vi "Read_Interlocks.vi"(8 "Error In":errorcluster, 11 "AccelNET.lvlib:TCP.lvclass":refnum<class "TCP.lvclass">) -> (0 "Error Out":errorcluster, 2 "Interlock Status":T1)   [LabVIEW 2012, in "AccelNET.lvlib" / "TCP.lvclass"]
uses:
  TCP.lvclass
  Interlocks.ctl
  Read_Selector.ctl
  Useful_Controls.lvlib
  Useful_SubVIs.lvlib
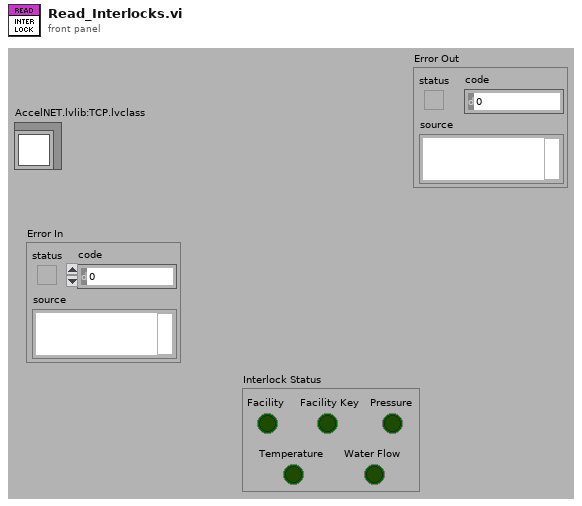
[diagram p1: front panel]
types:
  T1 = typedef "AccelNET.lvlib/Useful_Controls.lvlib/Interlocks.ctl" = cluster{"Facility":bool, "Facility Key":bool, "Water Flow":bool, "Pressure":bool, "Temperature":bool}
  T2 = typedef "AccelNET.lvlib/Useful_Controls.lvlib/Read_Selector.ctl" = u16
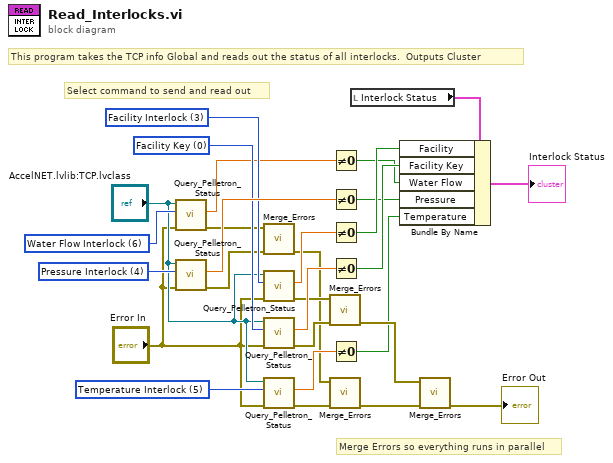
[diagram p0: block diagram]
diagram:
  w20 = T2 5 items=["Facility Key", "Chain Bypass", "Rotating Shaft Bypass", "Facility Interlock", "Pressure Interlock", "Temperature Interlock", "Water Flow Interlock", "Blower Status", "High Voltage", "+ High Voltage PS Readout", "- High Voltage PS Readout", "High Voltage PS Setting", "Ion Gauge", "Ion Filament", "Control Reference Voltage", "Control Mode", "Power Supply", "Chain Current", "Column Current", "Lost Current", "High Voltage Power Supply", "Rotating Shaft", "Chain", "Beamline GV"] ("Read Selector")
  w22 = T2 6 items=["Facility Key", "Chain Bypass", "Rotating Shaft Bypass", "Facility Interlock", "Pressure Interlock", "Temperature Interlock", "Water Flow Interlock", "Blower Status", "High Voltage", "+ High Voltage PS Readout", "- High Voltage PS Readout", "High Voltage PS Setting", "Ion Gauge", "Ion Filament", "Control Reference Voltage", "Control Mode", "Power Supply", "Chain Current", "Column Current", "Lost Current", "High Voltage Power Supply", "Rotating Shaft", "Chain", "Beamline GV"] ("Read Selector")
  w24 = T2 0 items=["Facility Key", "Chain Bypass", "Rotating Shaft Bypass", "Facility Interlock", "Pressure Interlock", "Temperature Interlock", "Water Flow Interlock", "Blower Status", "High Voltage", "+ High Voltage PS Readout", "- High Voltage PS Readout", "High Voltage PS Setting", "Ion Gauge", "Ion Filament", "Control Reference Voltage", "Control Mode", "Power Supply", "Chain Current", "Column Current", "Lost Current", "High Voltage Power Supply", "Rotating Shaft", "Chain", "Beamline GV"] ("Read Selector")
  w26 = T2 3 items=["Facility Key", "Chain Bypass", "Rotating Shaft Bypass", "Facility Interlock", "Pressure Interlock", "Temperature Interlock", "Water Flow Interlock", "Blower Status", "High Voltage", "+ High Voltage PS Readout", "- High Voltage PS Readout", "High Voltage PS Setting", "Ion Gauge", "Ion Filament", "Control Reference Voltage", "Control Mode", "Power Supply", "Chain Current", "Column Current", "Lost Current", "High Voltage Power Supply", "Rotating Shaft", "Chain", "Beamline GV"] ("Read Selector")
  w28 = T2 4 items=["Facility Key", "Chain Bypass", "Rotating Shaft Bypass", "Facility Interlock", "Pressure Interlock", "Temperature Interlock", "Water Flow Interlock", "Blower Status", "High Voltage", "+ High Voltage PS Readout", "- High Voltage PS Readout", "High Voltage PS Setting", "Ion Gauge", "Ion Filament", "Control Reference Voltage", "Control Mode", "Power Supply", "Chain Current", "Column Current", "Lost Current", "High Voltage Power Supply", "Rotating Shaft", "Chain", "Beamline GV"] ("Read Selector")
  # "Merge Errors so everything runs in parallel"
  # "Select command to send and read out"
  # "This program takes the TCP info Global and reads out the status of all interlocks.  Outputs Cluster"
  n1 = call "Query_Pelletron_Status.vi"("error in (no error)"="Error In", "Read Selector"=w22, "AccelNET.lvlib:TCP.lvclass"="AccelNET.lvlib:TCP.lvclass") -> ("error out"=w15:errorcluster, "Data Out"=w21:dbl)  [unwired: 7 in]
  n2 = call "Query_Pelletron_Status.vi"("error in (no error)"="Error In", "Read Selector"=w28, "AccelNET.lvlib:TCP.lvclass"="AccelNET.lvlib:TCP.lvclass") -> ("error out"=w14:errorcluster, "Data Out"=w27:dbl)  [unwired: 7 in]
  n3 = call "Merge_Errors.vi"("Error 2"=w14, "Error 1"=w15) -> ("Error Out"=w12:errorcluster)  [unwired: 9 in]
  n4 = call "Query_Pelletron_Status.vi"("error in (no error)"="Error In", "Read Selector"=w26, "AccelNET.lvlib:TCP.lvclass"="AccelNET.lvlib:TCP.lvclass") -> ("error out"=w17:errorcluster, "Data Out"=w25:dbl)  [unwired: 7 in]
  n5 = call "Query_Pelletron_Status.vi"("error in (no error)"="Error In", "Read Selector"=w24, "AccelNET.lvlib:TCP.lvclass"="AccelNET.lvlib:TCP.lvclass") -> ("error out"=w16:errorcluster, "Data Out"=w23:dbl)  [unwired: 7 in]
  n6 = call "Query_Pelletron_Status.vi"("error in (no error)"="Error In", "Read Selector"=w20, "AccelNET.lvlib:TCP.lvclass"="AccelNET.lvlib:TCP.lvclass") -> ("error out"=w13:errorcluster, "Data Out"=w19:dbl)  [unwired: 7 in]
  n7 = call "Merge_Errors.vi"("Error 2"=w16, "Error 1"=w17) -> ("Error Out"=w10:errorcluster)  [unwired: 9 in]
  n8 = call "Merge_Errors.vi"("Error 2"=w13, "Error 1"=w12) -> ("Error Out"=w11:errorcluster)  [unwired: 9 in]
  n9 = Not Equal To 0?(x=w21) -> (x != 0?=w5:bool)
  n10 = Not Equal To 0?(x=w27) -> (x != 0?=w4:bool)
  n11 = Not Equal To 0?(x=w25) -> (x != 0?=w7:bool)
  n12 = Not Equal To 0?(x=w23) -> (x != 0?=w6:bool)
  n13 = Not Equal To 0?(x=w19) -> (x != 0?=w3:bool)
  n14 = local read "Interlock Status"() -> (w1:T1)
  n15 = Bundle By Name(cluster=w1, "Facility"=w7, "Facility Key"=w6, "Water Flow"=w5, "Pressure"=w4, "Temperature"=w3) -> (→"Interlock Status":T1)
  n16 = call "Merge_Errors.vi"("Error 2"=w11, "Error 1"=w10) -> ("Error Out"=→"Error Out":errorcluster)  [unwired: 9 in]
